vi "noToCoord.vi"(2 "Pixel number":u16) -> (6 "i":u8, 7 "j":u8)   [LabVIEW 2019]
panel:
  in  "n(default:16)":u8=16
  in  "m (default:16)":u8=16
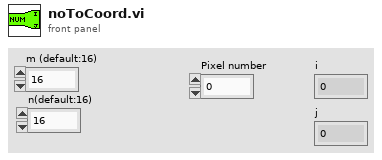
[diagram p1: front panel]
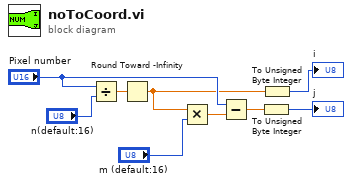
[diagram p0: block diagram]
diagram:
  n1 = Divide(x="Pixel number", y="n(default:16)") -> (x/y=w8:dbl)
  n2 = Round Toward -Infinity(1:w8) -> (0:w2:dbl)
  n3 = Multiply(x=w2, y="m (default:16)") -> (x*y=w6:dbl)
  n4 = Subtract(x="Pixel number", y=w6) -> (x-y=w4:dbl)
  n5 = To Unsigned Byte Integer(number=w4) -> (unsigned 8bit integer=→"j":u8)
  n6 = To Unsigned Byte Integer(number=w2) -> (unsigned 8bit integer=→"i":u8)
